vi "12-1.vi"() -> ()   [LabVIEW 2022 SP3, in "AoC22.lvlib"]
uses:
  AoC22.lvlib
  Map.ctl
panel:
  in  "Speed":u32(slide)
  out "Cur":cluster{"Row":i32, "Col":i32}
  out "Viz":i32[][](graph)
  out "Numeric":i32
  out "End gScore":i32
  out "Finished":bool
  out "No Solution":bool
  out "Elev":u8[][](graph)
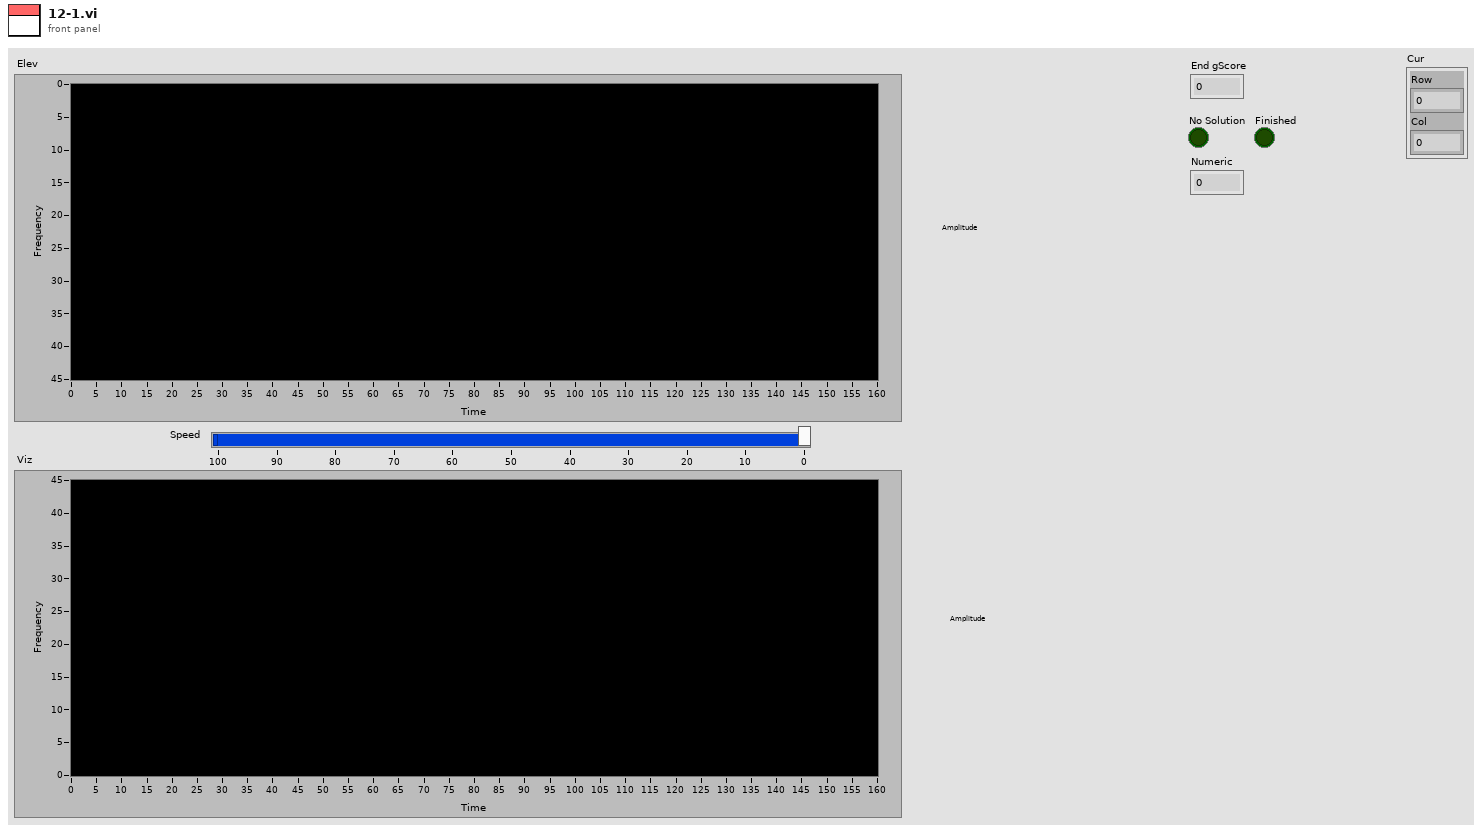
[diagram p1: front panel]
types:
  T1 = typedef "AoC22.lvlib/Map.ctl" = cluster{"Elevation":u8[][], "From":cluster{"Row":i32, "Col":i32}[][], "fScore":i32[][], "gScore":i32[][], "Start":cluster{"Row":i32, "Col":i32}, "End":cluster{"Row":i32, "Col":i32}, "openMap":map{i32, cluster{"Row":i32, "Col":i32}[]}, "openSet":set{cluster{"Row":i32, "Col":i32}}, "Vis":u8[][], "In Open":bool[][]}
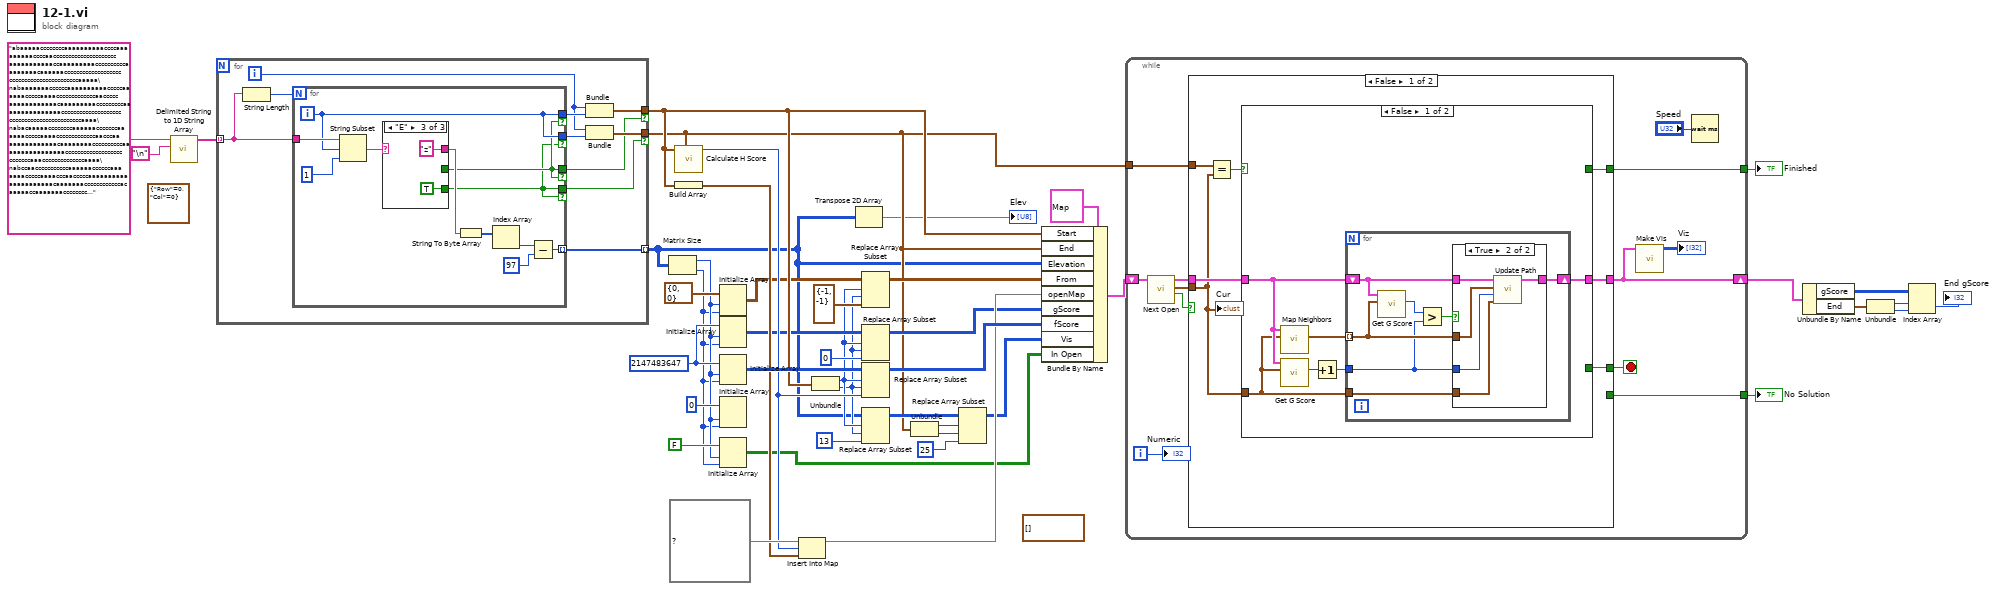
[diagram p0: block diagram]
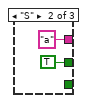
[diagram p3: hidden frame]
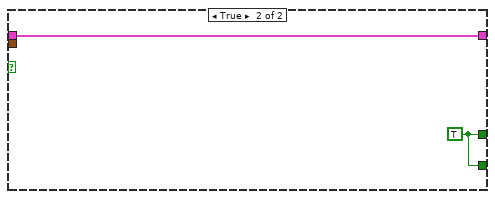
[diagram p6: hidden frame]
diagram:
  (unwired) cluster{"Row":i32, "Col":i32}[] [] ("Start")
  w35 = 2147483647 ("element")
  (unwired) cluster{"Row":i32, "Col":i32} {"Row"=0, "Col"=0}
  n1 = call <vilib>:"Delimited String to 1D String Array.vi"("delimiter"="\n", "delimited string"="abaaaaaccccccccaaaaaaaaaaccccaaaaaaaaaccccaacccccccccccccccccccccaaaaaaaaaaaccaaaaaaaaaccccccccccaaaaaaaacaaaaaaccccccccccccccccccccccccccccccccccccccccccaaaaa\nabaaaaaaaccccccaaaaaaaaaacccccaaaaaacccccaaaacccccccccccccaacccccaaaaaaaaaaaacaaaaaaaaacccccccccaaaaaaaaaaaaaaaccccccccccccccccccccccccccccccccccccccccccccaaaa\nabacaaaaaccccccccaaaaaacccccccaaaaaacccccaaaacccccccccccccaacccaaaaaaaaaaaaaacaaaaaaaaccccccccccaaaaaaaaaaaaaaaaccccccccccccccccccccccccccaaaccccccccccccccaaaa\nabccaacccccccccccaaaaaaccccccaaaaaaacccccaaaacccaacccccaaaaaaaaaaaaaaaaaaaaacaaaaaaaccccccccccccacaaaaaccaaaaaaacccccccc...") -> ("string array"=w42:string[])  [unwired: 9 in]
  n2 = for {
    tunnel: w42 -> [w53] mode=indexing
    tunnel: [w52] -> w5 mode=indexing
    tunnel: [w48] -> w32 if=w46
    tunnel: [w47] -> w10 if=w45
    i -> [w49]
    n3 = String Length(string=w53) -> (length=w54:i32)
    n4 = for {
      N: w54 -> [_]
      tunnel: w53 -> [w65]
      tunnel: [w61] -> w51 if=w60
      tunnel: [w60] -> w46 if=w60
      tunnel: [w59] -> w45 if=w59
      tunnel: [w61] -> w50 if=w59
      tunnel: [w55] -> w52 mode=indexing
      i -> [w61]
      n5 = String Subset(string=w65, offset (0)=w61, length (rest)=1 ("length (rest)")) -> (substring=w63:string)
      n6 = case shown="\"E\"" w63 {
        selector: w63 -> [w66 _ _]
        tunnel: [w66 "a" "z"] -> w62
        tunnel: [_ TRUE _] -> w60
        tunnel: [_ _ TRUE] -> w59
        frame Default {
        }
        frame "S" {
        }
        frame "E" {
        }
      }
      n7 = String To Byte Array(string=w62) -> (unsigned byte array=w58:u8[])
      n8 = Index Array(array=w58) -> (element=w57:u8)  [unwired: 1 in]
      n9 = Subtract(x=w57, y=u8 97) -> (x-y=w55:u8)
    }
    n10 = Bundle(w49, w51) -> (w48:cluster{i32, i32})  [unwired: 1 in]
    n11 = Bundle(w49, w50) -> (w47:cluster{i32, i32})  [unwired: 1 in]
  }
  n12 = Matrix Size(0:w5) -> (1:w3:i32, 2:w2:i32)
  n13 = call "Calculate H Score.vi"("End"=w10, "Position"=w32) -> ("hScore"=w31:i32)  [unwired: 9 in]
  n14 = Build Array(w32) -> (w33:cluster{i32, i32}[])
  n15 = Initialize Array(cluster{"Row":i32, "Col":i32} {"Row"=0, "Col"=0} ("Start"), w3, w2) -> (w27:cluster{"Row":i32, "Col":i32}[][])
  n16 = Initialize Array(w35, w3, w2) -> (w18:i32[][])
  n17 = Initialize Array(w35, w3, w2) -> (w38:i32[][])
  n18 = Initialize Array(u8 0 ("element"), w3, w2) -> ()  [unwired: 1 out]
  n19 = Initialize Array(FALSE, w3, w2) -> (w1:bool[][])
  n20 = Insert Into Map(map in=map{i32, cluster{"Row":i32, "Col":i32}[]} {} ("openSet"), key=w31, value=w33) -> (map out=w30:map{i32, cluster{"Row":i32, "Col":i32}[]})  [unwired: 2 out]
  n21 = Unbundle(w32) -> (w15:i32, w14:i32)
  n22 = Transpose 2D Array(2D array=w5) -> (transposed array=→"Elev":u8[][])
  n23 = Replace Array Subset(array=w27, new element=cluster{"Row":i32, "Col":i32} {"Row"=-1, "Col"=-1} ("new element/subarray"), index (row)=w15, index (col)=w14) -> (w28:cluster{"Row":i32, "Col":i32}[][])
  n24 = Replace Array Subset(array=w18, new element=0 ("new element/subarray"), index (row)=w15, index (col)=w14) -> (w19:i32[][])
  n25 = Replace Array Subset(array=w38, new element=w31, index (row)=w15, index (col)=w14) -> (w34:i32[][])
  n26 = Replace Array Subset(array=w5, new element=u8 13 ("new element/subarray"), index (row)=w15, index (col)=w14) -> (w12:u8[][])
  n27 = Unbundle(w10) -> (w9:i32, w8:i32)
  n28 = Replace Array Subset(array=w12, new element=u8 25 ("new element/subarray"), index (row)=w9, index (col)=w8) -> (w11:u8[][])
  n29 = Bundle By Name(cluster=T1 {"Elevation"=[], "From"=[], "fScore"=[], "gScore"=[], "Start"={"Row"=0, "Col"=0}, "End"={"Row"=0, "Col"=0}, "openMap"={}, "openSet"={}, "Vis"=[], "In Open"=[]} ("Map"), "Start"=w32, "End"=w10, "Elevation"=w5, "From"=w28, "openMap"=w30, "gScore"=w19, "fScore"=w34, "Vis"=w11, "In Open"=w1) -> (w37:T1)
  n30 = while {
    shift-right: [w72] -> w25
    shift-left: w37 -> [w82]
    tunnel: [w77] -> w36
    tunnel: w10 -> [w76]
    tunnel: [w75] -> w29
    i -> [w74]
    stop <- w78 stop-if-true
    n31 = call "Next Open.vi"("Map In"=w82) -> ("Empty?"=w81:bool, "Position"=w80:cluster{"Row":i32, "Col":i32}, "Map"=w79:T1)  [unwired: 8 in]
    n32 = case shown="False" w81 {
      tunnel: w80 -> [w83 _]
      tunnel: w79 -> [w87 w112]
      tunnel: [w84 w111] -> w78
      tunnel: [w85 w112] -> w72
      tunnel: [_ w111] -> w77
      tunnel: w76 -> [w89 _]
      tunnel: [w86 _] -> w75
      frame False {
        n33 = Equal?(x=w89, y=w83) -> (x = y?=w88:bool)
        n34 = case shown="False" w88 {
          selector: w88 -> [_ w109]
          tunnel: w87 -> [w94 w110]
          tunnel: [_ w109] -> w86
          tunnel: [w90 w110] -> w85
          tunnel: [_ w109] -> w84
          tunnel: w83 -> [w91 _]
          frame False {
            n35 = call "Map Neighbors.vi"("Position"=w91, "Map"=w94) -> ("Neighbors"=w95:cluster{"Row":i32, "Col":i32}[])  [unwired: 9 in]
            n36 = call "Get G Score.vi"("Position"=w91, "Map"=w94) -> ("gScore"=w93:i32)  [unwired: 9 in]
            n37 = Increment(x=w93) -> (x+1=w92:i32)
            n38 = for {
              shift-right: [w97] -> w90
              shift-left: w94 -> [w98]
              tunnel: w95 -> [w100] mode=indexing
              tunnel: w92 -> [w96]
              tunnel: w91 -> [w99]
              n39 = call "Get G Score.vi"("Position"=w100, "Map"=w98) -> ("gScore"=w102:i32)  [unwired: 9 in]
              n40 = Greater?(x=w102, y=w96) -> (0:w101:bool)
              n41 = case shown="True" w101 {
                tunnel: w100 -> [_ w107]
                tunnel: w99 -> [_ w105]
                tunnel: w98 -> [w103 w108]
                tunnel: [w103 w104] -> w97
                tunnel: w96 -> [_ w106]
                frame False {
                }
                frame True {
                  n42 = call "Update Path.vi"("From"=w105, "gScore"=w106, "Position"=w107, "Map In"=w108) -> ("Map"=w104:T1)  [unwired: 7 in]
                }
              }
            }
          }
          frame True {
          }
        }
        "Cur" <- w83
      }
      frame True {
        w111 = TRUE
      }
    }
    n43 = call "Make Vis.vi"("Map"=w72) -> ("Vis"=→"Viz":i32[][])  [unwired: 10 in]
    n44 = Wait (ms)(milliseconds to wait="Speed") -> ()  [unwired: 1 out]
    "Numeric" <- w74
  }
  "No Solution" <- w36
  "Finished" <- w29
  n45 = Unbundle By Name(w25) -> ("gScore"=w23:i32[][], "End"=w24:cluster{"Row":i32, "Col":i32})
  n46 = Unbundle(w24) -> ("Row"=w22:i32, "Col"=w21:i32)
  n47 = Index Array(array=w23, index (row)=w22, index (col)=w21) -> (element=→"End gScore":i32)
